vi "RGB Depth To Depth Array.vi"(1 "RGB Image":T1) -> (0 "Depth Array":u16[][](array[numeric]))   [LabVIEW 2018]
uses:
  <vilib>/vision/Image Controls.llb/IMAQ Image.ctl
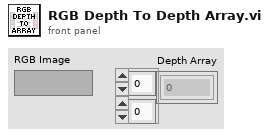
[diagram p1: front panel]
types:
  T1 = typedef "IMAQ Image.ctl" = refnum<image>
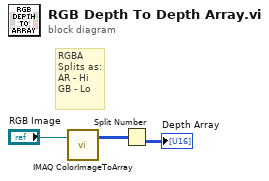
[diagram p0: block diagram]
diagram:
  # "RGBA\nSplits as:\nAR - Hi\nGB - Lo"
  n1 = call "IMAQ ColorImageToArray"("Image"="RGB Image") -> ("Image Pixels (U32)"=w2:u32[][])  [unwired: 3 in, 2 out]
  n2 = Split Number(x=w2) -> (lo(x)=→"Depth Array":u16[][])  [unwired: 1 out]
